vi "氨氮总磷加标回收 (子VI).vi"(11 "是否启动对话框":bool) -> ()   [LabVIEW 2016, in "质控单元.lvlib"]
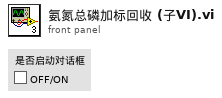
[diagram p1: front panel]
types:
  T1 = cluster{"是否启用仪器":bool, "CODMn":cluster{"启动测量模式":cluster{"测量模式":enum16{"水样测量", "标样核查", "加标回收", "平行样", "校零", "校标"}}, "确定按钮":bool}, "启动模块":cluster{"氨氮":bool, "总磷":bool, "总氮":bool, "CODMn":bool, "CODCr":bool}, "常规启动":bool, "直接启动":bool}
  T2 = enum32{"Bad", "Idle", "Run top level", "Running"}
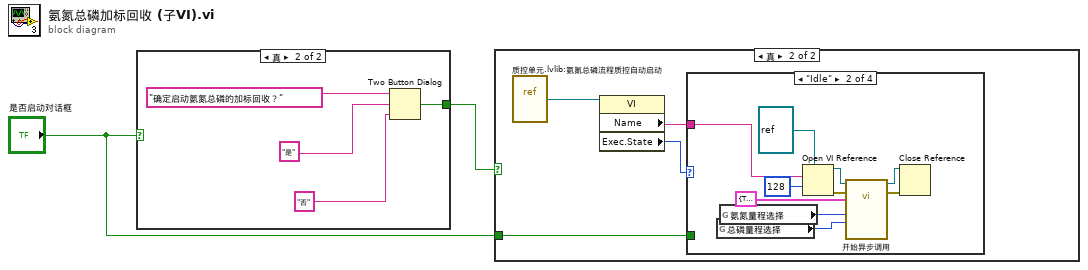
[diagram p0: block diagram]
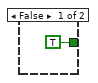
[diagram p2: hidden frame]
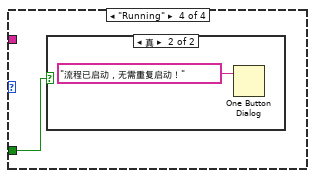
[diagram p6: hidden frame]
diagram:
  n1 = case shown="真" "是否启动对话框" {
    tunnel: [TRUE ("T button?") w7] -> w2
    frame False {
    }
    frame True {
      n2 = Two Button Dialog(message="确定启动氨氮总磷的加标回收？" ("消息"), 1:"否" ("F按钮名称（“取消”）"), 2:"是" ("T按钮名称（“确定”）")) -> (T button?=w7:bool)
    }
  }
  n3 = case shown="真" w2 {
    tunnel: "是否启动对话框" -> [_ w8]
    frame False {
    }
    frame True {
      n4 = vi-ref "质控单元.lvlib:氨氮总磷流程质控自动启动.vi"() -> (w11:refnum<vi>)
      n5 = property class="VI"(reference=w11) -> ("Name"=w9:string, "Exec.State"=w10:T2)  [unwired: 1 in, 2 out]
      n6 = case shown="\"Idle\"" w10 {
        tunnel: w9 -> [_ w17 _ _]
        tunnel: w8 -> [_ _ _ w22]
        frame "Bad", Default {
        }
        frame "Idle" {
          n7 = global read "断电保存全局.vi" "总磷量程选择"() -> (w13:enum32{"H", "L", "AUTO"})
          n8 = global read "断电保存全局.vi" "氨氮量程选择"() -> (w14:enum32{"H", "L", "AUTO"})
          n9 = Open VI Reference(type specifier VI Refnum (for type only)=refnum<vi> refnum ("类型说明符VI引用句柄（仅用于类型）"), vi path=w17, options=128 ("选项")) -> (vi reference=w21:refnum<vi>, error out=w16:errorcluster)  [unwired: 3 in]
          n10 = call-by-ref "开始异步调用"(reference=w21, error in=w16, "总磷量程切换"=w13, "氨氮量程切换"=w14, "参数"=T1 {"是否启用仪器"=TRUE, "CODMn"={"启动测量模式"={"测量模式"=enum."水样测量"}, "确定按钮"=FALSE}, "启动模块"={"氨氮"=TRUE, "总磷"=TRUE, "总氮"=FALSE, "CODMn"=FALSE, "CODCr"=FALSE}, "常规启动"=FALSE, "直接启动"=TRUE}) -> (reference out=w20:refnum<vi>, error out=w15:errorcluster)  [unwired: 9 in]
          n11 = Close Reference(reference=w20, error in (no error)=w15) -> ()  [unwired: 1 out]
        }
        frame "Run top level" {
        }
        frame "Running" {
          n12 = case shown="真" w22 {
            frame False {
            }
            frame True {
              n13 = One Button Dialog(message="流程已启动，无需重复启动！" ("消息")) -> ()  [unwired: 1 in, 1 out]
            }
          }
        }
      }
    }
  }
